vi "Generate Event.vi"(4 "Actions":T2, 6 "Origin":string, 7 "Classification":T1, 8 "Error In":errorcluster, 9 "Comment":string, 10 "Description":string, 11 "EventLog in":refnum<class "EventLog.lvclass">) -> (0 "Error Out":errorcluster, 3 "Events out":refnum<class "Event.lvclass">)   [LabVIEW 2019, in "Event.lvclass"]
uses:
  Event.lvclass
  SubModules/EventLog/EventLog.lvclass
  EventsAbstract/TypeDef/Event Actions.ctl
  Modules/ModuleAbstract/ModuleAbstract/TypeDef/Module Actions.ctl
  <vilib>/ActorFramework/Message Enqueuer/Message Enqueuer.lvclass
  TypeDef/Event Classification.ctl
  Event.lvclass/Event.ctl
  EventsAbstract/EventsAbstract.lvclass
  Modules/ModuleAbstract/ModuleAbstract/ModuleAbstract.lvclass
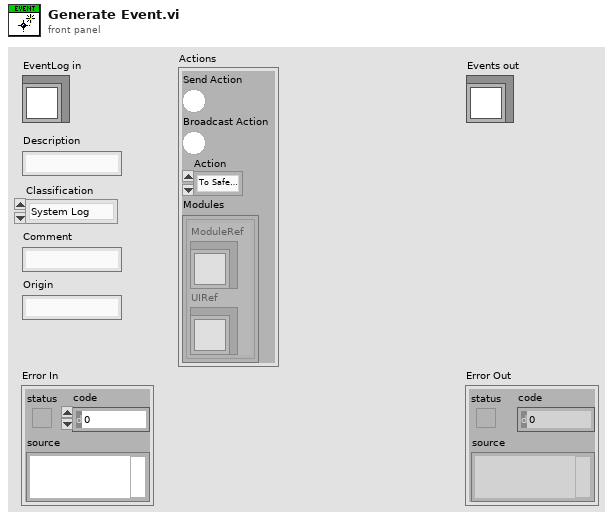
[diagram p1: front panel]
types:
  T1 = typedef "Event.lvclass/Event Classification.ctl" = enum16{"System Log"}
  T2 = typedef "EventsAbstract.lvclass/Event Actions.ctl" = cluster{"Send Action":bool, "Broadcast Action":bool, "Action":T3, "Modules":cluster{"ModuleRef":refnum<class "Message Enqueuer.lvclass">, "UIRef":refnum<class "Message Enqueuer.lvclass">}[]}
  T3 = typedef "ModuleAbstract.lvlib/ModuleAbstract.lvclass/Module Actions.ctl" = enum16{"To Safe State", "Reset Safe State", "Close Module"}
  T4 = cluster{"Date":string, "Time":string, "Description":string, "Comments":string, "Origin":string}
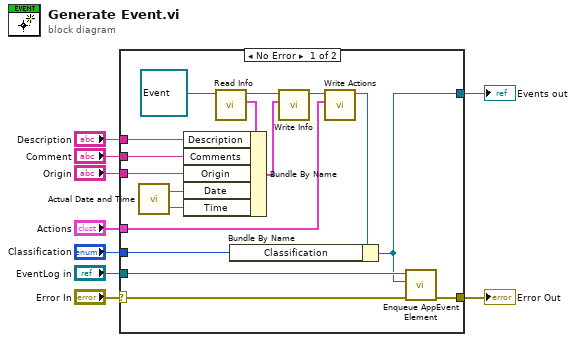
[diagram p0: block diagram]
diagram:
  n1 = case shown="No Error" "Error In" {
    selector: "Error In" -> [w26 w27]
    tunnel: [w25 w27] -> w4
    tunnel: [w11 _] -> w5
    tunnel: "Description" -> [w20 _]
    tunnel: "Comment" -> [w19 _]
    tunnel: "EventLog in" -> [w24 _]
    tunnel: "Actions" -> [w13 _]
    tunnel: "Origin" -> [w18 _]
    tunnel: "Classification" -> [w10 _]
    frame No Error {
      n2 = call "Actual Date and Time.vi"() -> ("Actual Time"=w16:string, "Actual Date"=w17:string)  [unwired: 2 in]
      n3 = call-dynamic "Read Info.vi"("EventsAbstract in"=refnum<class "Event.lvclass"> refnum ("Events.lvclass")) -> ("Info"=w22:T4, "EventsAbstract out"=w21:refnum<class "Event.lvclass">)  [unwired: 8 in, 1 out]
      n4 = Bundle By Name(cluster=w22, "Description"=w20, "Comments"=w19, "Origin"=w18, "Date"=w17, "Time"=w16) -> (w15:T4)
      n5 = call-dynamic "Write Info.vi"("Info"=w15, "EventsAbstract in"=w21) -> ("EventsAbstract out"=w14:refnum<class "Event.lvclass">)  [unwired: 8 in, 1 out]
      n6 = call-dynamic "Write Actions.vi"("Actions"=w13, "EventsAbstract in"=w14) -> ("EventsAbstract out"=w12:refnum<class "Event.lvclass">)  [unwired: 8 in, 1 out]
      n7 = Bundle By Name(cluster=w12, "Classification"=w10) -> (w11:refnum<class "Event.lvclass">)
      n8 = call "Enqueue AppEvent Element.vi"("Error In"=w26, "Event Occured"=w11, "EventLog in"=w24) -> ("Error Out"=w25:errorcluster)  [unwired: 6 in, 2 out]
    }
    frame Error {
    }
  }
  "Error Out" <- w4
  "Events out" <- w5
